vi "state change logic BAP4B.vi"(1 "mode set":T1, 2 "system state in":T2={"last light state"=enum."init", "light state"=enum."go EW", "state time (ms)"=10000, "current time (ms)"=0, "time remaining (ms)"=10000, "change state"=FALSE}, 11 "exit":bool) -> (3 "system state out":T2={"last light state"=enum."left turn E", "light state"=enum."go EW", "state time (ms)"=54295007, "current time (ms)"=4706, "time remaining (ms)"=54290301, "change state"=TRUE}, 8 "change state":bool=TRUE, 15 "exit program":bool)   [LabVIEW 2014]
doc: "state change logic BAP4B\n\nManages which of the three modes: automatic, blinking, or all on is executed as the set light values and updates the system state. This takes into account the exit button, state and current time from system, and its mode set.\n \nBeverly Abadines\nPHY 350\nP4"
uses:
  typedefs/system state cluster.ctl
  typedefs/state enum.ctl
  typedefs/control mode enum.ctl
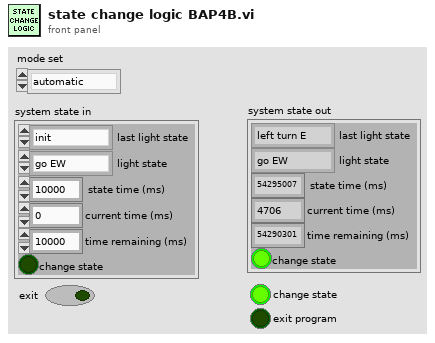
[diagram p1: front panel]
types:
  T1 = typedef "control mode enum.ctl" = enum16{"automatic", "blinking", "all on test"}
  T2 = typedef "system state cluster.ctl" = cluster{"last light state":T3, "light state":T3, "state time (ms)":i32, "current time (ms)":i32, "time remaining (ms)":i32, "change state":bool}
  T3 = typedef "state enum.ctl" = enum16{"init", "idle", "left turn E", "go EW", "caution EW", "left turn W", "left turn N", "go NS", "caution NS", "left turn S", "blink on", "blink off", "all on test", "exit"}
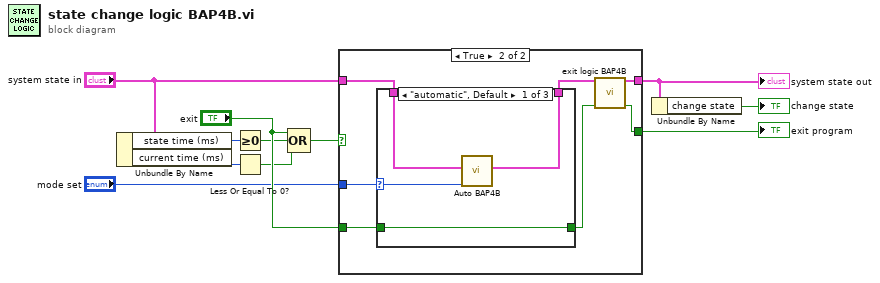
[diagram p0: block diagram]
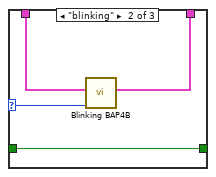
[diagram p3: hidden frame]
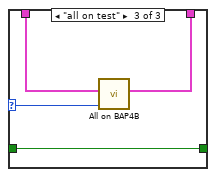
[diagram p4: hidden frame]
diagram:
  n1 = Unbundle By Name("system state in") -> ("state time (ms)"=w3:i32, "current time (ms)"=w2:i32)
  n2 = Greater Or Equal To 0?(x=w3) -> (x >= 0?=w4:bool)
  n3 = Less Or Equal To 0?(x=w2) -> (x <= 0?=w1:bool)
  n4 = Compound Arithmetic op=OR("exit", w4, w1) -> (w11:bool)
  n5 = case shown="True" w11 {
    tunnel: [_ w19] -> w8
    tunnel: [w12 w18] -> w10
    tunnel: "system state in" -> [w12 w14]
    tunnel: "exit" -> [_ w17]
    tunnel: "mode set" -> [_ w15]
    frame False {
    }
    frame True {
      n6 = case shown="\"automatic\", Default" w15 {
        selector: w15 -> [w23 w26 w31]
        tunnel: [w20 w27 w28] -> w16
        tunnel: w17 -> [w20 w27 w28]
        tunnel: w14 -> [w22 w25 w30]
        tunnel: [w21 w24 w29] -> w13
        frame "automatic", Default {
          n7 = call "Auto BAP4B.vi"("mode set"=w23, "system state in"=w22) -> ("system state out"=w21:T2)  [unwired: 9 in]
        }
        frame "blinking" {
          n8 = call "Blinking BAP4B.vi"("mode set"=w26, "system state in"=w25) -> ("system state out"=w24:T2)  [unwired: 9 in]
        }
        frame "all on test" {
          n9 = call "All on BAP4B.vi"("mode set"=w31, "system state in"=w30) -> ("system state out"=w29:T2)  [unwired: 9 in]
        }
      }
      n10 = call "exit logic BAP4B.vi"("system state in"=w13, "exit"=w16) -> ("system state out"=w18:T2, "exit program"=w19:bool)  [unwired: 12 in]
    }
  }
  "system state out" <- w10
  "exit program" <- w8
  n11 = Unbundle By Name(w10) -> ("change state"=→"change state":bool)
